vi "CSM - Convert Error to Argument.vi"(4 "Error":errorcluster) -> (1 "Argument":string)   [LabVIEW 2017, in "Communicable State Machine.lvlib"]
doc: "Converts a LabVIEW Error Cluster to the CSM error argument format.\n\n> [!NOTE] \n> <b>CSM Argument Type</b>\n>\n> In CSM, all arguments and return values are presented in string format, but they can carry any data type underneath. Therefore, the sender must encode first, and the receiver must decode afterwards. For example, CSM has a built-in HEXSTR encoding scheme, and custom codecs can also be extended as needed. To facilitate the identification of the encoding method, it is recommended to write the encoded argument in the format `<Argument Type> STRING FORMAT ARGUMENT`. Use the CSM - Argument Type VI to extract the type tag and select the corresponding decoding function accordingly.\n\n> [!NOTE] \n> <b>CSM ERRSTR Format Argument</b>\n>\n> The LabVIEW Error Cluster is a complex data type. The error information string usually contains carriage returns, which cannot be directly passed as a CSM argument. Although error cluster information can be converted to HEXSTR format, this method lacks readability, making it impossible to read information intuitively in logs. Therefore, to pass LabVIEW error information in CSM arguments, CSM has a built-in ERRSTR format argument encoding/decoding scheme. The argument type string is ERRSTR. The conversion process is as follows:\n>\n> 1. Format the code and source in the error cluster into a string with the following format: \n>\n> Error: `<ERRSTR>[Error: error-code] error-description-As-safe-argument-string`\n> Warning: `<ERRSTR>[Warning: error-code] warning-description-As-safe-argument-string`\n>\n> 2. Replace special characters in this string with safe characters.\n>\n> 3. Obtain the CSM ERRSTR format argument, which can be safely embedded in the state string without disrupting CSM message parsing.\n\n\n<b>Reference Example</b>: `[CSM-Example]\\0. Base Concepts\\4.2 Arguments - Error As Arguments.vi`.\n\n-- <b>Controls</b> --\n- <b>Error</b>: LabVIEW Error Cluster.\n\n-- <b>Indicators</b> --\n- <b>Argument</b>: CSM error argument format."
uses:
  Communicable State Machine.lvlib
  CSM - Keywords.vi
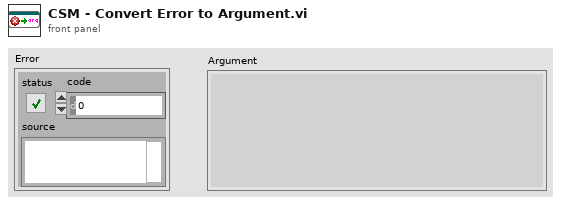
[diagram p1: front panel]
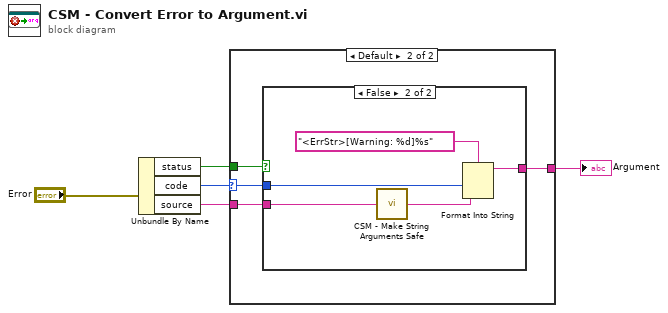
[diagram p0: block diagram]
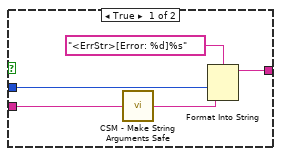
[diagram p3: hidden frame]
diagram:
  n1 = Unbundle By Name("Error") -> ("status"=w1:bool, "code"=w3:i32, "source"=w2:string)
  n2 = case shown="Default" w3 {
    selector: w3 -> [_ w8]
    tunnel: [_ w9] -> w5
    tunnel: w2 -> [_ w7]
    tunnel: w1 -> [_ w6]
    frame 0 {
    }
    frame Default {
      n3 = case shown="False" w6 {
        tunnel: [w14 w19] -> w9
        tunnel: w8 -> [w11 w16]
        tunnel: w7 -> [w10 w15]
        frame True {
          n4 = call "CSM - Make String Arguments Safe.vi"("Argument String"=w10) -> ("Safe Argument String"=w12:string)  [unwired: 8 in]
          n5 = Format Into String(format string="<ErrStr>[Error: %d]%s", w11, w12) -> (resulting string=w14:string)  [unwired: 2 in, 1 out]
        }
        frame False {
          n6 = call "CSM - Make String Arguments Safe.vi"("Argument String"=w15) -> ("Safe Argument String"=w17:string)  [unwired: 8 in]
          n7 = Format Into String(format string="<ErrStr>[Warning: %d]%s", w16, w17) -> (resulting string=w19:string)  [unwired: 2 in, 1 out]
        }
      }
    }
  }
  "Argument" <- w5
